vi "Run Sequence.vi"() -> ()   [LabVIEW 2019, in "Run Sequence.lvlib"]
uses:
  Run Sequence.lvlib
  support/States.ctl
  support/StateData.ctl
  <vilib>/Utility/miscctls.llb/LVRowAndColumnTypeDef.ctl
  <vilib>/Utility/sysdir.llb/System Directory Type.ctl
  <vilib>/Utility/file.llb/Read Delimited Spreadsheet (string).vi
  <vilib>/Utility/file.llb/Write Delimited Spreadsheet (string).vi
panel:
  in  "Open Sequences Folder":bool
  out "Sequence":string[][](table)
  in  "Select Sequence":i32(listbox)=-1
  in  "Run Sequence":bool
  # "Run Sequence"
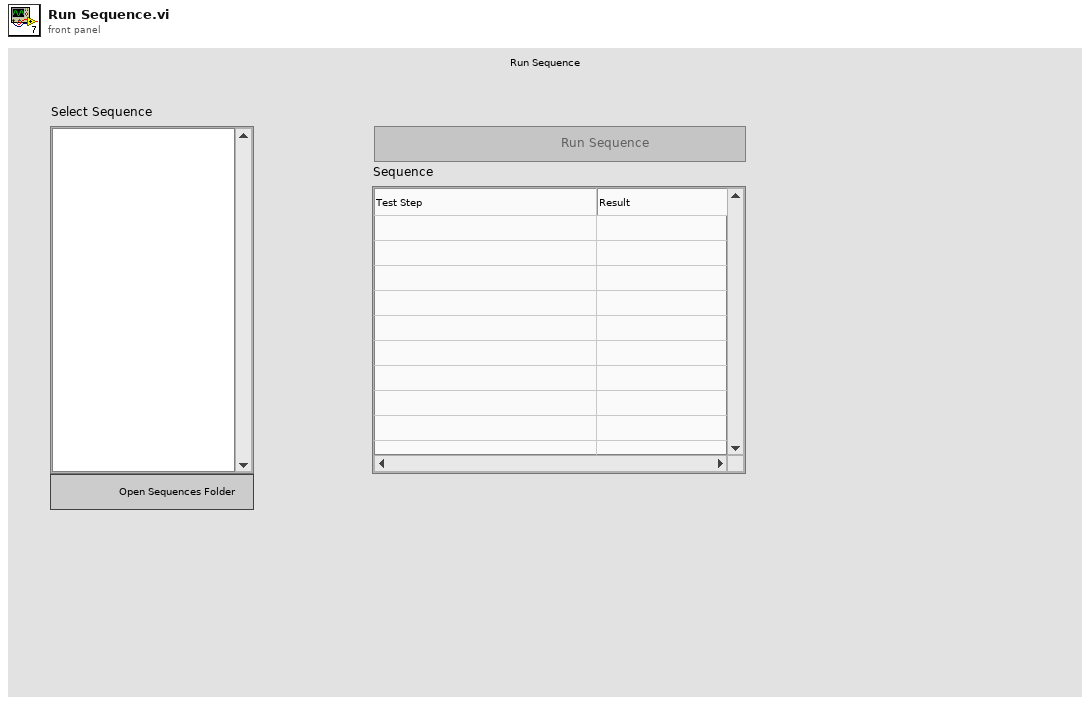
[diagram p1: front panel]
types:
  T1 = typedef "Run Sequence.lvlib/StateData.ctl" = cluster{"Sequence filepaths":path[], "Sequence table":string[][], "Sequence name":string, "Reports folder":path, "Sequences folder":path}
  T2 = typedef "Run Sequence.lvlib/States.ctl" = enum16{"Initialize", "Wait for Event", "Run Sequence", "Log Report File", "Shutdown"}
  T3 = typedef "LVRowAndColumnTypeDef.ctl" = cluster{"Row":i32, "Column":i32}
  T4 = enum8{"Enabled", "Disabled", "Disabled and Grayed Out"}
  T5 = typedef "System Directory Type.ctl" = i32
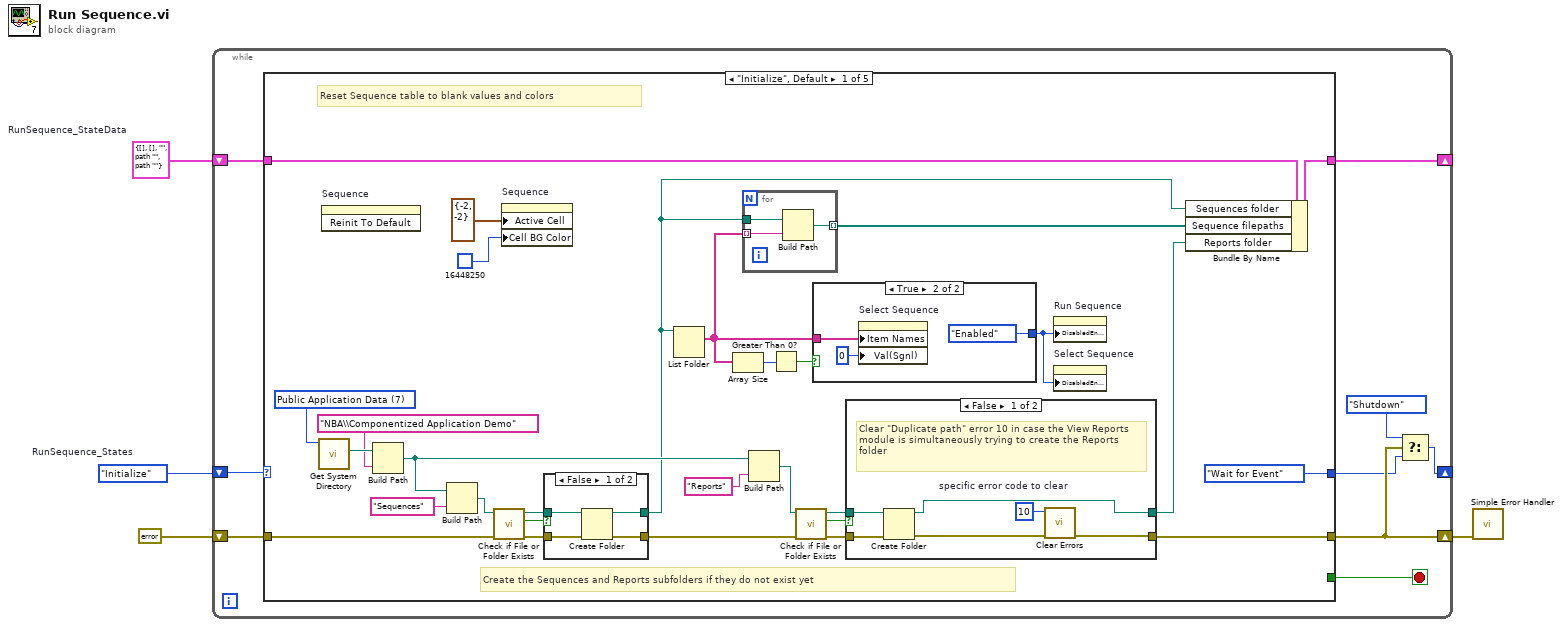
[diagram p0: block diagram]
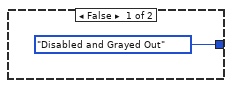
[diagram p2: hidden frame]
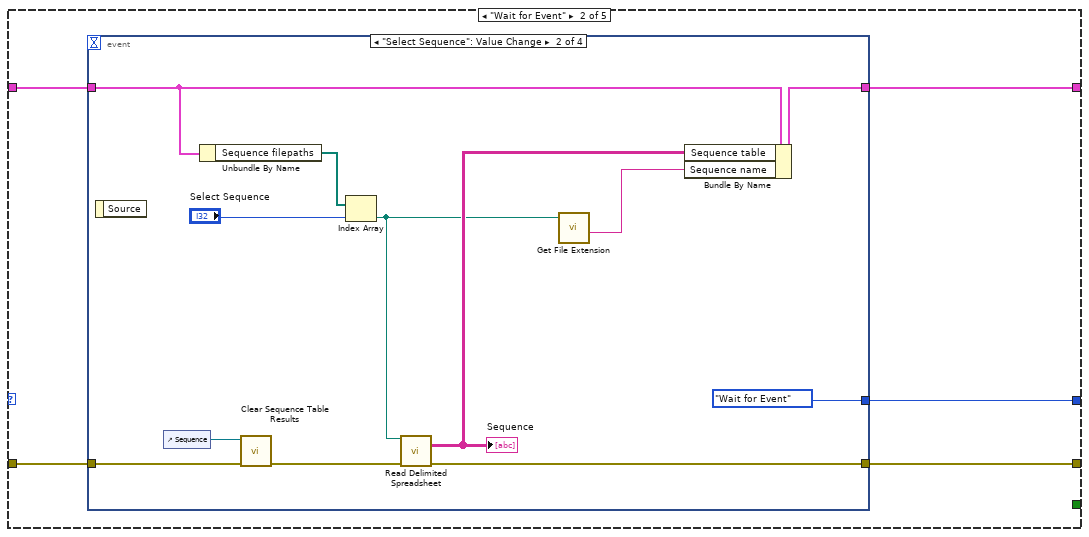
[diagram p5: hidden frame]
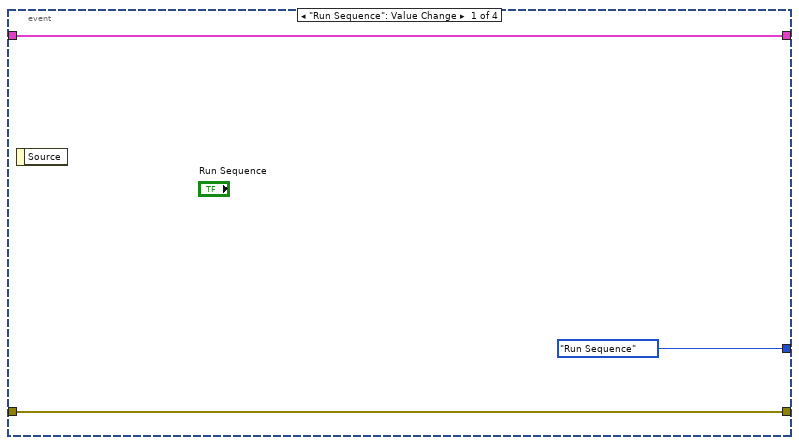
[diagram p6: hidden frame]
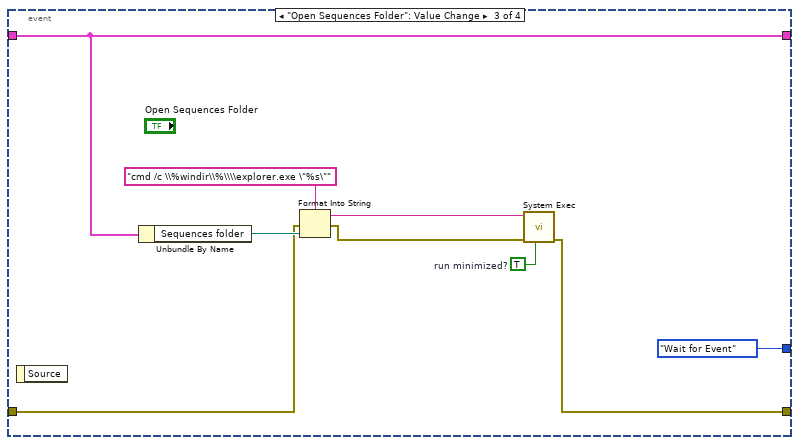
[diagram p7: hidden frame]
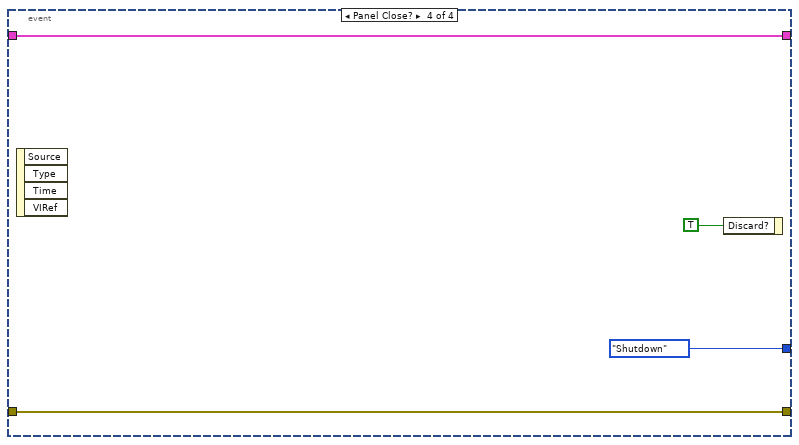
[diagram p8: hidden frame]
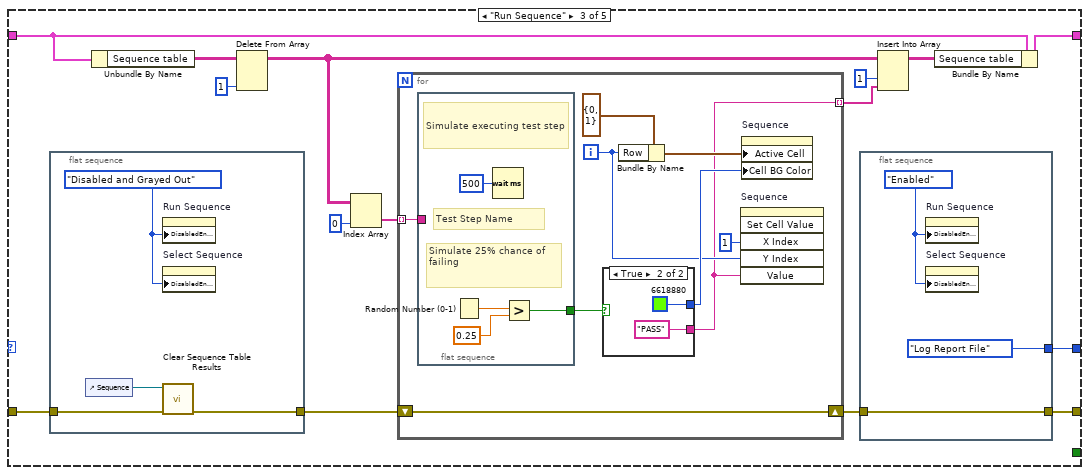
[diagram p9: hidden frame]
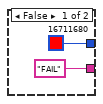
[diagram p10: hidden frame]
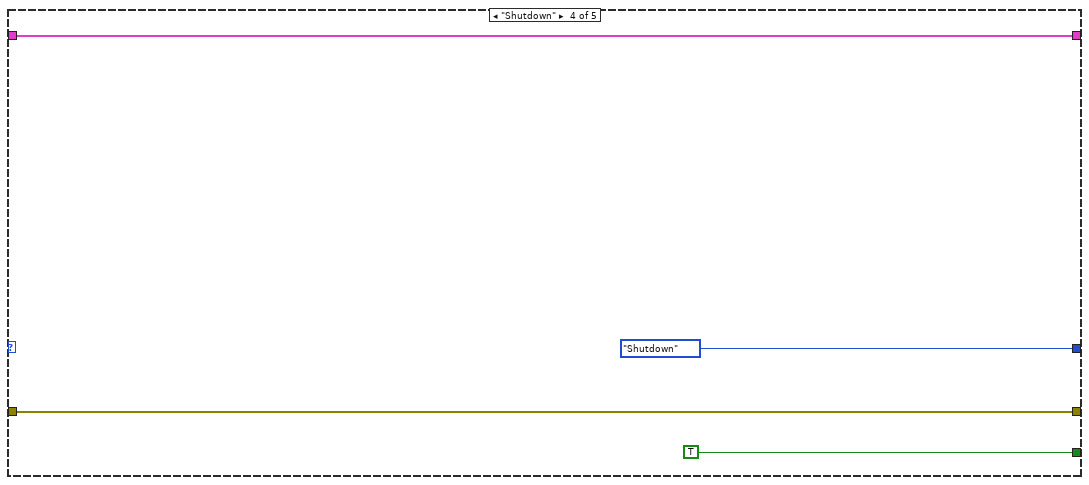
[diagram p11: hidden frame]
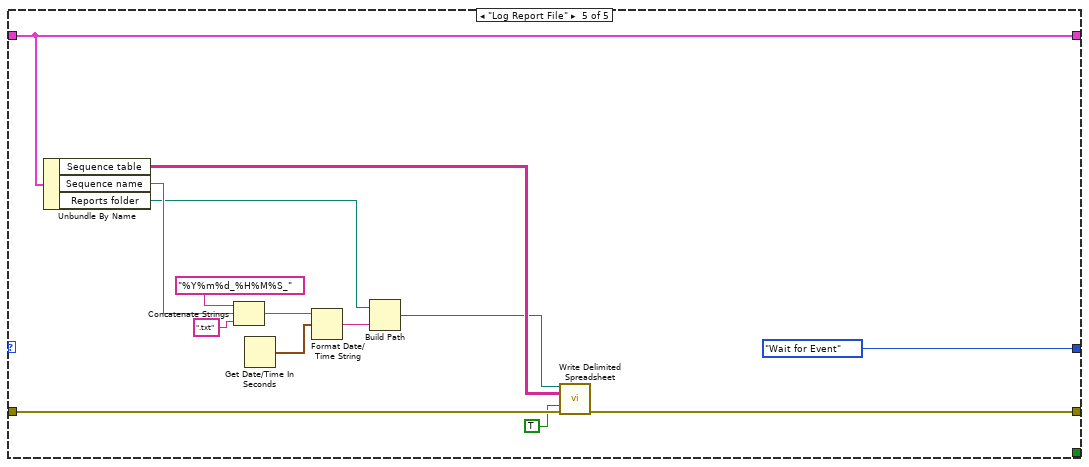
[diagram p12: hidden frame]
diagram:
  w3 = T1 {"Sequence filepaths"=[], "Sequence table"=[], "Sequence name"="", "Reports folder"=path "", "Sequences folder"=path ""}  # RunSequence_StateData
  w4 = States."Initialize"  # RunSequence_States
  n1 = while {
    shift-right: [w5] -> _
    shift-left: w4 -> [w13]
    shift-right: [w11] -> _
    shift-left: w3 -> [w12]
    shift-right: [w8] -> w1
    shift-left: errorcluster {"status"=FALSE, "code"=0, "source"=""} ("error in (no error)") -> [w9]
    stop <- w10 stop-if-true
    n2 = case shown="\"Initialize\", Default" w13 {
      tunnel: [States."Wait for Event" w68 w106 States."Shutdown" States."Wait for Event"] -> w7
      tunnel: w12 -> [w40 w67 w111 w139 w152]
      tunnel: [w39 w66 w102 w139 w152] -> w11
      tunnel: [_ _ _ TRUE _] -> w10
      tunnel: w9 -> [w25 w65 w108 w136 w153]
      tunnel: [w33 w64 w104 w136 w149] -> w8
      frame "Initialize", Default {
        w30 = T5 7 items=["User Home"=0, "User Desktop"=1, "User Documents"=2, "User Application Data"=3, "User Preferences"=4, "User Temporary"=5, "Public Documents"=6, "Public Application Data"=7, "Public Preferences"=8, "Public Cache"=13, "System Core Libraries"=9, "System Installed Libraries"=10, "Application Files"=11, "Boot Volume Root"=12] ("system directory type")
        # "Create the Sequences and Reports subfolders if they do not exist yet"
        # "Reset Sequence table to blank values and colors"
        n3 = call <vilib>:"Get System Directory.vi"("system directory type"=w30) -> ("system directory"=w22:path)  [unwired: 10 in]
        n4 = invoke on="Sequence" class="Tbl (strict)" method="Reinit To Default"() -> ()  [unwired: 3 in, 3 out]
        n5 = Build Path(base path=w22, name or relative path="NBA\\Componentized Application Demo") -> (appended path=w20:path)
        n6 = Build Path(base path=w20, name or relative path="Sequences") -> (appended path=w24:path)
        n7 = call <vilib>:"Check if File or Folder Exists.vi"("error in (no error)"=w25, "path"=w24) -> ("error out"=w26:errorcluster, "file or folder exists?"=w27:bool, "dup path"=w28:path)  [unwired: 7 in]
        n8 = property on="Sequence" class="Tbl (strict)"("Active Cell"=T3 {"Row"=-2, "Column"=-2} ("Active Cell:Active Cell"), "Cell BG Color"=u32 16448250) -> ()  [unwired: 2 in, 2 out]
        n9 = case shown="False" w27 {
          tunnel: w26 -> [w49 w52]
          tunnel: [w50 w52] -> w23
          tunnel: w28 -> [w48 w51]
          tunnel: [w47 w51] -> w14
          frame False {
            n10 = Create Folder(path (use dialog)=w48, error in=w49) -> (created path=w47:path, error out=w50:errorcluster)  [unwired: 1 in, 1 out]
          }
          frame True {
          }
        }
        n11 = List Folder(path=w14) -> (filenames=w19:string[])  [unwired: 3 in, 3 out]
        n12 = Array Size(array=w19) -> (size(s)=w18:i32)
        n13 = for {
          tunnel: w14 -> [w63]
          tunnel: w19 -> [w62] mode=indexing
          tunnel: [w61] -> w38 mode=indexing
          n14 = Build Path(base path=w63, name or relative path=w62) -> (appended path=w61:path)
        }
        n15 = Build Path(base path=w20, name or relative path="Reports") -> (appended path=w35:path)
        n16 = Greater Than 0?(x=w18) -> (x > 0?=w17:bool)
        n17 = call <vilib>:"Check if File or Folder Exists.vi"("error in (no error)"=w23, "path"=w35) -> ("error out"=w34:errorcluster, "file or folder exists?"=w32:bool, "dup path"=w31:path)  [unwired: 7 in]
        n18 = case shown="True" w17 {
          tunnel: w19 -> [_ w45]
          tunnel: [T4."Disabled and Grayed Out" ("Disabled") T4."Enabled" ("Disabled")] -> w16
          frame False {
          }
          frame True {
            n19 = property on="Select Sequence" class="LstBox (strict)"("Item Names"=w45, "Val(Sgnl)"=0 ("Select Sequence")) -> ()  [unwired: 2 in, 2 out]
          }
        }
        n20 = case shown="False" w32 {
          tunnel: w34 -> [w58 w60]
          tunnel: [w53 w60] -> w33
          tunnel: w31 -> [w57 w59]
          tunnel: [w56 w59] -> w15
          frame False {
            w55 = 10  # specific error code to clear
            # "Clear \"Duplicate path\" error 10 in case the View Reports module is simultaneously trying to create the Reports folder"
            n21 = Create Folder(path (use dialog)=w57, error in=w58) -> (created path=w56:path, error out=w54:errorcluster)  [unwired: 1 in, 1 out]
            n22 = call <vilib>:"Clear Errors.vi"("error in (no error)"=w54, "specific error code to clear (0: all)"=w55) -> ("error out"=w53:errorcluster)  [unwired: 4 in, 1 out]
          }
          frame True {
          }
        }
        n23 = property on="Run Sequence" class="Bool"("DisabledEnum"=w16) -> ()  [unwired: 2 in, 2 out]
        n24 = property on="Select Sequence" class="LstBox (strict)"("DisabledEnum"=w16) -> ()  [unwired: 2 in, 2 out]
        n25 = Bundle By Name(cluster=w40, "Sequences folder"=w14, "Sequence filepaths"=w38, "Reports folder"=w15) -> (w39:T1)
      }
      frame "Wait for Event" {
        n26 = event shown="[1] \"Select Sequence\": Value Change" {
          selector: _ -> [_ _ _ _]
          dyn-events: _ -> [_ _ _ _]
          timeout: _ -> [_ _ _ _]
          tunnel: [States."Run Sequence" States."Wait for Event" States."Wait for Event" States."Shutdown"] -> w68
          tunnel: w67 -> [w70 w83 w87 w94]
          tunnel: [w70 w78 w87 w94] -> w66
          tunnel: w65 -> [w69 w75 w86 w93]
          tunnel: [w69 w74 w85 w93] -> w64
          event "Run Sequence": Value Change {
            n27 = event-data() -> ()  [unwired: 1 in, 1 out]
          }
          event "Select Sequence": Value Change {
            n28 = event-data() -> ()  [unwired: 1 in, 1 out]
            n29 = control-ref of="Sequence"() -> (w77:refnum<vi>)
            n30 = Unbundle By Name(w83) -> ("Sequence filepaths"=w82:path[])
            n31 = call "Clear Sequence Table Results.vi"("error in (no error)"=w75, "table reference in"=w77) -> ("error out"=w76:errorcluster)  [unwired: 8 in, 1 out]
            n32 = Index Array(array=w82, index="Select Sequence") -> (element=w73:path)
            n33 = call-poly <vilib>:"Read Delimited Spreadsheet.vi"("file path (dialog if empty)"=w73, "error in (no error)"=w76) -> ("all rows"=w79:string[][], "error out"=w74:errorcluster)  [unwired: 8 in, 4 out]
            "Sequence" <- w79
            n34 = call <vilib>:"Get File Extension.vi"("file"=w73) -> ("filename without extension"=w72:string)  [unwired: 6 in, 4 out]
            n35 = Bundle By Name(cluster=w83, "Sequence table"=w79, "Sequence name"=w72) -> (w78:T1)
          }
          event "Open Sequences Folder": Value Change {
            w90 = TRUE  # run minimized?
            n36 = event-data() -> ()  [unwired: 1 in, 1 out]
            n37 = Unbundle By Name(w87) -> ("Sequences folder"=w89:path)
            n38 = Format Into String(format string="cmd /c \\%windir\\%\\\\explorer.exe \"%s\"" ("name or relative path"), error in=w86, w89) -> (resulting string=w91:string, error out=w88:errorcluster)  [unwired: 1 in]
            n39 = call <vilib>:"System Exec.vi"("run minimized? (F)"=w90, "error in (no error)"=w88, "command line"=w91) -> ("error out"=w85:errorcluster)  [unwired: 5 in, 3 out]
          }
          event Panel Close? {
            n40 = event-data() -> ()  [unwired: 1 in, 4 out]
            n41 = event-data("Discard?"=TRUE) -> ()  [unwired: 1 in, 1 out]
          }
        }
      }
      frame "Run Sequence" {
        n42 = flat-sequence {
          tunnel: w108 -> [w116]
          tunnel: [w115] -> w107
          frame #0 {
            w118 = T4."Disabled and Grayed Out" ("Disabled")
            n43 = control-ref of="Sequence"() -> (w117:refnum<vi>)
            n44 = property on="Run Sequence" class="Bool"("DisabledEnum"=w118) -> ()  [unwired: 2 in, 2 out]
            n45 = property on="Select Sequence" class="LstBox (strict)"("DisabledEnum"=w118) -> ()  [unwired: 2 in, 2 out]
            n46 = call "Clear Sequence Table Results.vi"("error in (no error)"=w116, "table reference in"=w117) -> ("error out"=w115:errorcluster)  [unwired: 8 in, 1 out]
          }
        }
        n47 = Unbundle By Name(w111) -> ("Sequence table"=w99:string[][])
        n48 = Delete From Array(array=w99, index (col)=1 ("disabled index (col)")) -> (array with subset deleted=w98:string[][])  [unwired: 2 in, 1 out]
        n49 = Index Array(array=w98, index (col)=0 ("disabled index (col)")) -> (element=w109:string[])  [unwired: 1 in]
        n50 = for {
          tunnel: w109 -> [w122] mode=indexing
          shift-right: [w120] -> w105
          shift-left: w107 -> [w120]
          tunnel: [w119] -> w103 mode=indexing
          i -> [w123]
          n51 = flat-sequence {
            tunnel: w122 -> [_]
            tunnel: [w128] -> w121
            frame #0 {
              # "Test Step Name"
              # "Simulate 25% chance of failing"
              # "Simulate executing test step"
              n52 = Random Number (0-1)() -> (number: 0 to 1=w130:dbl)
              n53 = Wait (ms)(milliseconds to wait=u32 500) -> ()  [unwired: 1 out]
              n54 = Greater?(x=w130, y=0.25) -> (0:w128:bool)
            }
          }
          n55 = case shown="True" w121 {
            tunnel: [u32 16711680 u32 6618880] -> w127
            tunnel: ["FAIL" ("Value") "PASS" ("Value")] -> w119
            frame False {
            }
            frame True {
            }
          }
          n56 = Bundle By Name(cluster=T3 {"Row"=0, "Column"=1} ("Active Cell:Active Cell"), "Row"=w123) -> (w125:T3)
          n57 = invoke on="Sequence" class="Tbl (strict)" method="Set Cell Value"("X Index"=1 ("Y Index"), "Y Index"=w123, "Value"=w119) -> ()  [unwired: 3 in, 6 out]
          n58 = property on="Sequence" class="Tbl (strict)"("Active Cell"=w125, "Cell BG Color"=w127) -> ()  [unwired: 2 in, 2 out]
        }
        n59 = flat-sequence {
          tunnel: [States."Log Report File"] -> w106
          tunnel: w105 -> [w112]
          tunnel: [w112] -> w104
          frame #0 {
            w114 = T4."Enabled" ("Disabled")
            n60 = property on="Run Sequence" class="Bool"("DisabledEnum"=w114) -> ()  [unwired: 2 in, 2 out]
            n61 = property on="Select Sequence" class="LstBox (strict)"("DisabledEnum"=w114) -> ()  [unwired: 2 in, 2 out]
          }
        }
        n62 = Insert Into Array(array=w98, index (col)=1 ("disabled index (col)"), new element=w103) -> (w101:string[][])  [unwired: 1 in]
        n63 = Bundle By Name(cluster=w111, "Sequence table"=w101) -> (w102:T1)
      }
      frame "Shutdown" {
      }
      frame "Log Report File" {
        n64 = Unbundle By Name(w152) -> ("Sequence table"=w148:string[][], "Sequence name"=w143:string, "Reports folder"=w140:path)
        n65 = Concatenate Strings("%Y%m%d_%H%M%S_" ("time format string (%c)"), w143, ".txt" ("element")) -> (w141:string)
        n66 = Get Date/Time In Seconds() -> (seconds since 1Jan1904=w151:timestamp)
        n67 = Format Date/Time String(time format string (%c)=w141, seconds (now)=w151) -> (date/time string=w150:string)  [unwired: 1 in]
        n68 = Build Path(base path=w140, name or relative path=w150) -> (appended path=w147:path)
        n69 = call-poly <vilib>:"Write Delimited Spreadsheet.vi"("file path (dialog if empty)"=w147, "2D data"=w148, "append to file? (new file:F)"=TRUE, "error in (no error)"=w153) -> ("error out"=w149:errorcluster)  [unwired: 10 in, 1 out]
      }
    }
    n70 = Select(t=States."Shutdown", s=w8, f=w7) -> (s? t:f=w5:T2)
  }
  n71 = call <vilib>:"Simple Error Handler.vi"("error in (no error)"=w1) -> ()  [unwired: 4 in, 5 out]
